vi "replace_bytes.vi"(9 "offset (-1: current position)":i32=-1, 10 "bytes to write":refnum<class "Bytes.lvclass">, 11 "Bytes in":refnum<class "Bytes.lvclass">) -> (3 "Bytes out":refnum<class "Bytes.lvclass">)   [LabVIEW 2020, in "lvdata.lvlib" / "Bytes.lvclass"]
uses:
  Bytes.lvclass
  Bytes.lvclass/Bytes.ctl
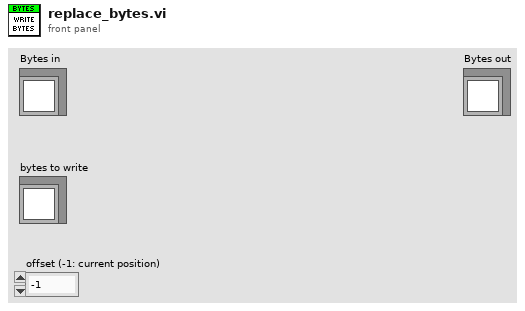
[diagram p1: front panel]
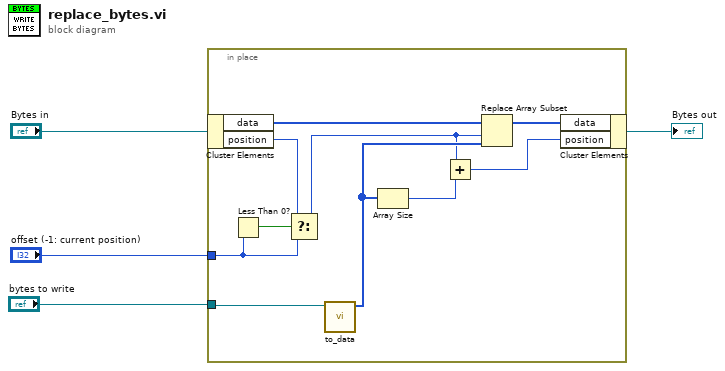
[diagram p0: block diagram]
diagram:
  n1 = in-place {
    in-place-border: "offset (-1: current position)" -> [w12]
    in-place-border: "bytes to write" -> [w11]
    n2 = in-place-cluster #1("Bytes in") -> ("data"=w9:u8[], "position"=w13:i32)
    n3 = Less Than 0?(x=w12) -> (x < 0?=w14:bool)
    n4 = Select(t=w13, s=w14, f=w12) -> (s? t:f=w7:i32)
    n5 = call "to_data.vi"("Bytes in"=w11) -> ("byte array"=w8:u8[])  [unwired: 10 in]
    n6 = Array Size(array=w8) -> (size(s)=w6:i32)
    n7 = Add(x=w7, y=w6) -> (x+y=w5:i32)
    n8 = Replace Array Subset(array=w9, new element=w8, index=w7) -> (w10:u8[])
    n9 = in-place-cluster #1("data"=w10, "position"=w5) -> (→"Bytes out":refnum<class "Bytes.lvclass">)
  }
